vi "Flatten.vi"(8 "error in":errorcluster, 9 "Data":T1) -> (0 "error out":errorcluster, 2 "Buffer":u8[](array[numeric]) format="%.0x")   [LabVIEW 2020, in "UdpPayload.lvlib"]
uses:
  UdpPayload.lvlib
  Data.ctl
  <vilib>/IlluminatedG/IG Protoc/LV-Proto/LV-Proto.lvlib
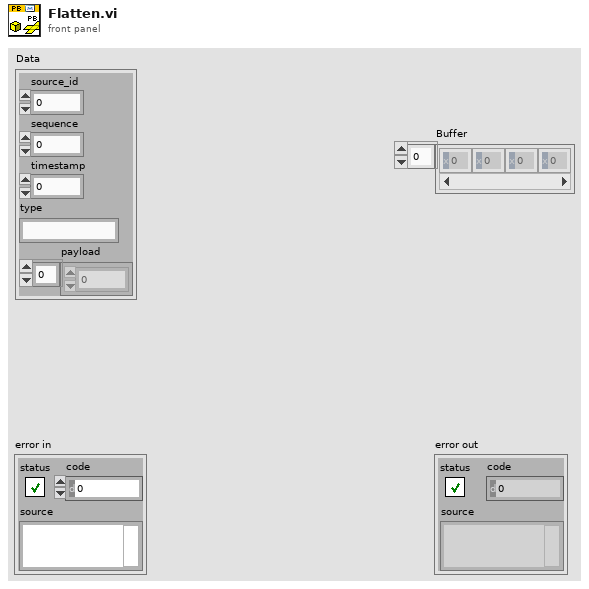
[diagram p1: front panel]
types:
  T1 = typedef "UdpPayload.lvlib/Data.ctl" = cluster{"source_id":u32, "sequence":u32, "timestamp":u64, "type":string, "payload":u8[]}
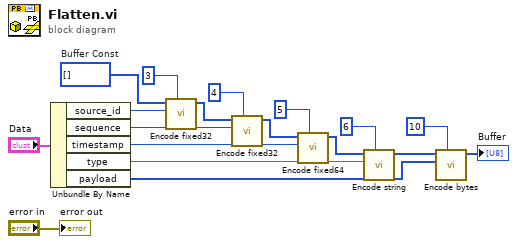
[diagram p0: block diagram]
diagram:
  w16 = u8[] []  # Buffer Const
  n1 = Unbundle By Name("Data") -> ("source_id"=w14:u32, "sequence"=w11:u32, "timestamp"=w8:u64, "type"=w5:string, "payload"=w2:u8[])
  n2 = call <vilib>:"Encode fixed32.vi"("Field Number"=3, "fixed32"=w14, "Buffer in"=w16) -> ("Buffer"=w13:u8[])  [unwired: 8 in]
  n3 = call <vilib>:"Encode fixed32.vi"("Field Number"=4, "fixed32"=w11, "Buffer in"=w13) -> ("Buffer"=w10:u8[])  [unwired: 8 in]
  n4 = call <vilib>:"Encode fixed64.vi"("Field Number"=5, "fixed64"=w8, "Buffer in"=w10) -> ("Buffer"=w7:u8[])  [unwired: 8 in]
  n5 = call <vilib>:"Encode string.vi"("Field Number"=6, "string"=w5, "Buffer in"=w7) -> ("Buffer"=w4:u8[])  [unwired: 8 in]
  n6 = call <vilib>:"Encode bytes.vi"("Field Number"=10, "bytes"=w2, "Buffer in"=w4) -> ("Buffer"=→"Buffer":u8[])  [unwired: 8 in]
  "error out" <- "error in"
